vi "ConfigDialog-WithoutLoadingModules.vi"(8 "error in (no error)":errorcluster, 11 "INI File Path":path) -> (0 "error out":errorcluster)   [LabVIEW 2018]
uses:
  NistPluggableModules/Sensor/SensorPlugins/SensorBaseClass/SensorBase.lvclass
  C:/Program Files (x86)/National Instruments/LabVIEW 2018/user.lib/NIST/BaseClasses/BasePlugin_class/BasePlugin.lvclass
  <userlib>/NIST/BaseClasses/BasePlugin_class/BasePlugin.lvclass/BasePlugin.ctl
  <userlib>/NIST/ModuleAdminLib/CloneRegistration/CloneRegistration.lvclass
  <userlib>/NIST/ModuleAdminLib/ModuleAdmin/Accessors/Read CloneRegRef.vi
  <userlib>/NIST/BaseClasses/BasePlugin_class/Accessors/Write PluginIniFilePath.vi
  NistPluggableModules/Sync/SyncModule/Main.vi
  NistPluggableModules/FGen/FgenModule/Main.vi
  NistPluggableModules/Analysis/AnalysisModule/Main.vi
  <vilib>/Utility/error.llb/Error Cluster From Error Code.vi
  <vilib>/ErrorRing/Error Ring.xnode
  <userlib>/NIST/ModuleAdminLib/ModuleAdmin/ModuleAdmin.lvclass
  NistPluggableModules/Sync/SyncModule/SyncModule.lvlib
  <userlib>/NIST/NISTErrorLib/NISTErrorLib.lvlib
  NistPluggableModules/FGen/FgenModule/FgenModule.lvlib
  NistPluggableModules/Digitizer/DigitizerModule/DigitizerModule.lvlib
  NistPluggableModules/Scope/ScopeModule/ScopeModule.lvlib
  NistPluggableModules/Scope/ScopeShared/ScopeShared.lvlib
  NistPluggableModules/Analysis/AnalysisModule/AnalysisModule.lvlib
  NistPluggableModules/AcPwr/AcPwrModule/AcPwrModule.lvlib
  NistPluggableModules/AcPwr/AcPwrShared/AcPwrShared.lvlib
panel:
  out "Changed":bool
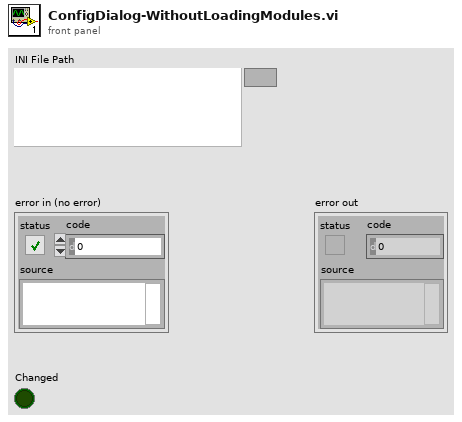
[diagram p1: front panel]
types:
  T1 = typedef "SyncModule.lvlib/clBroadcastEvents.ctl" = cluster{"DidInit":refnum<user-event>, "StatusUpdate":refnum<user-event>, "ErrorReport":refnum<user-event>, "DidStop":refnum<user-event>, "PathToINI":refnum<user-event>, "TriggerTime":refnum<user-event>, "LockStatus":refnum<user-event>, "Info":refnum<user-event>, "ClockProperties":refnum<user-event>}
  T2 = typedef "FgenModule.lvlib/clBroadcastEvents.ctl" = cluster{"DidInit":refnum<user-event>, "StatusUpdate":refnum<user-event>, "ErrorReport":refnum<user-event>, "DidStop":refnum<user-event>, "PathToINI":refnum<user-event>, "Channels":refnum<user-event>, "Function":refnum<user-event>, "Waveforms":refnum<user-event>, "Triggers":refnum<user-event>, "FunctionParams":refnum<user-event>, "FunctionArbs":refnum<user-event>, "FunctionSampleRate":refnum<user-event>}
  T3 = typedef "DigitizerShared.lvlib/clBroadcastEvents.ctl" = cluster{"DidInit":refnum<user-event>, "StatusUpdate":refnum<user-event>, "ErrorReport":refnum<user-event>, "DidStop":refnum<user-event>, "PathToINI":refnum<user-event>, "Channels":refnum<user-event>, "Acq":refnum<user-event>, "Trigger":refnum<user-event>, "Waveforms":refnum<user-event>}
  T4 = typedef "ScopeShared.lvlib/clBroadcastEvents.ctl" = cluster{"DidInit":refnum<user-event>, "StatusUpdate":refnum<user-event>, "ErrorReport":refnum<user-event>, "DidStop":refnum<user-event>, "PathToINI":refnum<user-event>, "Handle":refnum<user-event>, "Model":refnum<user-event>, "Channels":refnum<user-event>, "Acquisition":refnum<user-event>, "Trigger":refnum<user-event>, "ExtAcquisition":refnum<user-event>, "Waveform":refnum<user-event>}
  T5 = typedef "AnalysisModule.lvlib/clBroadcastEvents.ctl" = cluster{"DidInit":refnum<user-event>, "StatusUpdate":refnum<user-event>, "ErrorReport":refnum<user-event>, "DidStop":refnum<user-event>, "PathToINI":refnum<user-event>, "Config":refnum<user-event>, "ResultReport":refnum<user-event>, "FunctionClass":refnum<user-event>, "State":refnum<user-event>, "FunctionParams":refnum<user-event>, "Duration":refnum<user-event>}
  T6 = typedef "AcPwrShared.lvlib/AcPwrBroadcastEvents.ctl" = cluster{"DidInit":refnum<user-event>, "StatusUpdate":refnum<user-event>, "ErrorReport":refnum<user-event>, "DidStop":refnum<user-event>, "PathToINI":refnum<user-event>, "Measurements":refnum<user-event>, "LoadConfigFile":refnum<user-event>, "GetSettings":refnum<user-event>, "SetSettings":refnum<user-event>, "GetType&ID":refnum<user-event>, "GotSettings":refnum<user-event>}
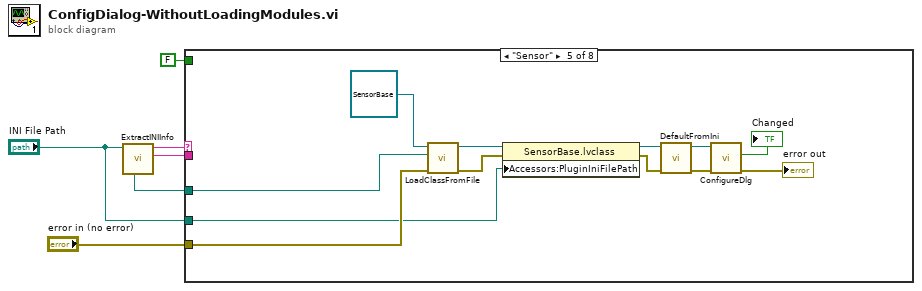
[diagram p0: block diagram]
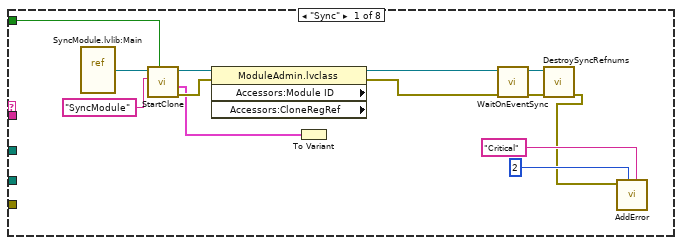
[diagram p2: hidden frame]
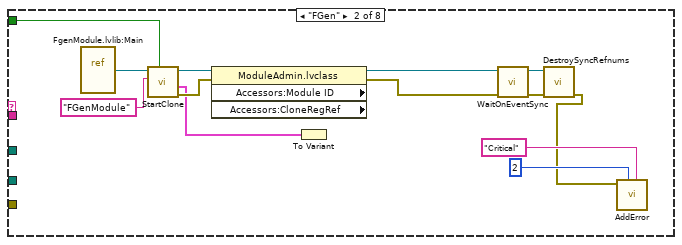
[diagram p3: hidden frame]
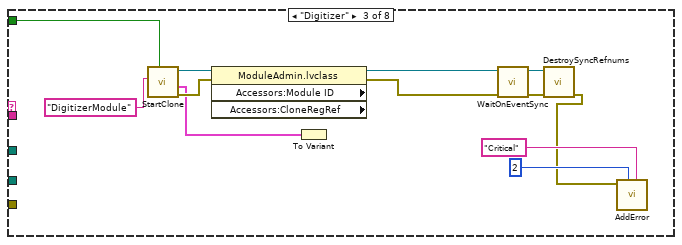
[diagram p4: hidden frame]
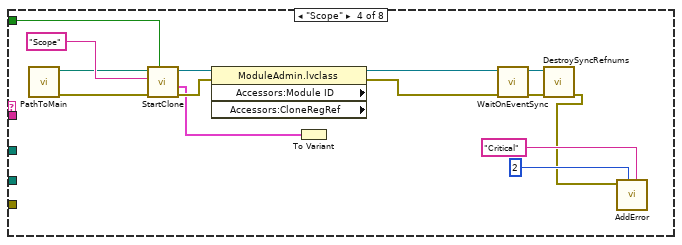
[diagram p5: hidden frame]
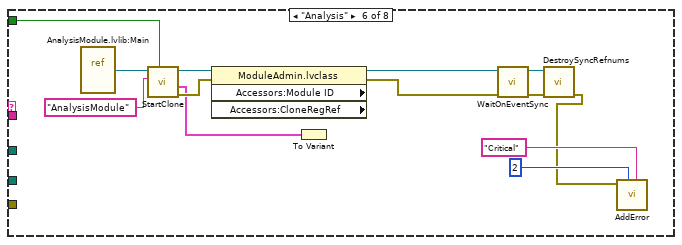
[diagram p6: hidden frame]
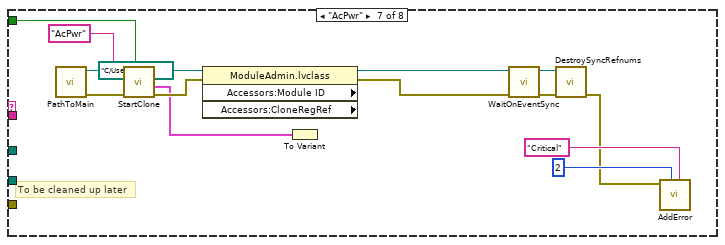
[diagram p7: hidden frame]
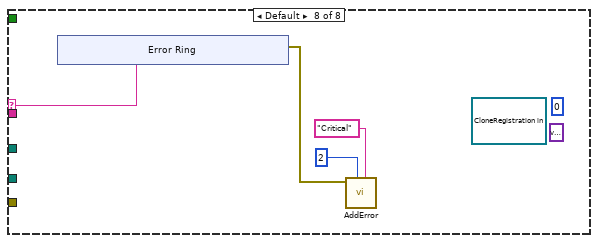
[diagram p8: hidden frame]
diagram:
  n1 = call "ExtractINIInfo.vi"("INI File Path"="INI File Path") -> ("Instrument name"=w4:string, "Module Name"=w6:string, "Instrument Class Path"=w1:path)  [unwired: 4 in, 4 out]
  n2 = case shown="\"Sensor\"" w6 {
    selector: w6 -> [_ _ _ _ _ _ _ w101]
    tunnel: FALSE ("ShowPanel? (f)") -> [w7 w20 w33 w47 _ w71 w86 _]
    tunnel: w4 -> [_ _ _ _ _ _ _ _]
    tunnel: "error in (no error)" -> [_ _ _ _ w68 _ _ _]
    tunnel: "INI File Path" -> [_ _ _ _ w65 _ _ _]
    tunnel: w1 -> [_ _ _ _ w59 _ _ _]
    frame "Sync" {
      n3 = vi-ref "SyncModule.lvlib:Main.vi"() -> (w19:refnum<vi>)
      n4 = call "StartClone.vi"("ShowPanel? (f)"=w7, "ModuleName"="SyncModule", "VI Refnum"=w19) -> ("error out"=w12:errorcluster, "SyncBroadcastEvents"=w11:T1, "ModuleAdmin"=w17:refnum<class "ModuleAdmin.lvclass">)  [unwired: 6 in]
      n5 = property class="ModuleAdmin.lvclass" props=["Accessors:Module ID", "Accessors:CloneRegRef"](reference=w17, error in=w12) -> (reference out=w15:refnum<class "ModuleAdmin.lvclass">, error out=w16:errorcluster)  [unwired: 2 out]
      n6 = To Variant(anything=w11) -> ()  [unwired: 1 out]
      n7 = call <userlib>:"WaitOnEventSync.vi"("error in (no error)"=w16, "ModuleAdmin"=w15) -> ("error out"=w14:errorcluster, "ModuleAdmin"=w13:refnum<class "ModuleAdmin.lvclass">)  [unwired: 8 in]
      n8 = call <userlib>:"DestroySyncRefnums.vi"("error in (no error)"=w14, "ModuleAdmin"=w13) -> ("error out"=w8:errorcluster)  [unwired: 9 in]
      n9 = call <userlib>:"AddError.vi"("Severity"="Critical", "Priority"=u8 2, "error in (no error)"=w8) -> ()  [unwired: 7 in, 2 out]
    }
    frame "FGen" {
      n10 = vi-ref "FgenModule.lvlib:Main.vi"() -> (w32:refnum<vi>)
      n11 = call "StartClone.vi"("ShowPanel? (f)"=w20, "ModuleName"="FGenModule", "VI Refnum"=w32) -> ("error out"=w25:errorcluster, "clBroadcastEvents"=w24:T2, "ModuleAdmin"=w30:refnum<class "ModuleAdmin.lvclass">)  [unwired: 6 in]
      n12 = property class="ModuleAdmin.lvclass" props=["Accessors:Module ID", "Accessors:CloneRegRef"](reference=w30, error in=w25) -> (reference out=w28:refnum<class "ModuleAdmin.lvclass">, error out=w29:errorcluster)  [unwired: 2 out]
      n13 = To Variant(anything=w24) -> ()  [unwired: 1 out]
      n14 = call <userlib>:"WaitOnEventSync.vi"("error in (no error)"=w29, "ModuleAdmin"=w28) -> ("error out"=w27:errorcluster, "ModuleAdmin"=w26:refnum<class "ModuleAdmin.lvclass">)  [unwired: 8 in]
      n15 = call <userlib>:"DestroySyncRefnums.vi"("error in (no error)"=w27, "ModuleAdmin"=w26) -> ("error out"=w21:errorcluster)  [unwired: 9 in]
      n16 = call <userlib>:"AddError.vi"("Severity"="Critical", "Priority"=u8 2, "error in (no error)"=w21) -> ()  [unwired: 7 in, 2 out]
    }
    frame "Digitizer" {
      n17 = call "StartClone.vi"("ShowPanel? (f)"=w33, "ModuleName"="DigitizerModule") -> ("error out"=w38:errorcluster, "clBroadcastEvents"=w37:T3, "ModuleAdmin"=w43:refnum<class "ModuleAdmin.lvclass">)  [unwired: 7 in]
      n18 = property class="ModuleAdmin.lvclass" props=["Accessors:Module ID", "Accessors:CloneRegRef"](reference=w43, error in=w38) -> (reference out=w41:refnum<class "ModuleAdmin.lvclass">, error out=w42:errorcluster)  [unwired: 2 out]
      n19 = To Variant(anything=w37) -> ()  [unwired: 1 out]
      n20 = call <userlib>:"WaitOnEventSync.vi"("error in (no error)"=w42, "ModuleAdmin"=w41) -> ("error out"=w40:errorcluster, "ModuleAdmin"=w39:refnum<class "ModuleAdmin.lvclass">)  [unwired: 8 in]
      n21 = call <userlib>:"DestroySyncRefnums.vi"("error in (no error)"=w40, "ModuleAdmin"=w39) -> ("error out"=w34:errorcluster)  [unwired: 9 in]
      n22 = call <userlib>:"AddError.vi"("Severity"="Critical", "Priority"=u8 2, "error in (no error)"=w34) -> ()  [unwired: 7 in, 2 out]
    }
    frame "Scope" {
      n23 = call "PathToMain.vi"() -> ("Error Out"=w46:errorcluster, "PathToMain"=w45:path)  [unwired: 10 in]
      n24 = call "StartClone.vi"("ShowPanel? (f)"=w47, "error in (no error)"=w46, "ModuleName"="Scope", "vi path"=w45) -> ("error out"=w52:errorcluster, "clBroadcastEvents"=w51:T4, "ModuleAdmin"=w57:refnum<class "ModuleAdmin.lvclass">)  [unwired: 5 in]
      n25 = property class="ModuleAdmin.lvclass" props=["Accessors:Module ID", "Accessors:CloneRegRef"](reference=w57, error in=w52) -> (reference out=w55:refnum<class "ModuleAdmin.lvclass">, error out=w56:errorcluster)  [unwired: 2 out]
      n26 = To Variant(anything=w51) -> ()  [unwired: 1 out]
      n27 = call <userlib>:"WaitOnEventSync.vi"("error in (no error)"=w56, "ModuleAdmin"=w55) -> ("error out"=w54:errorcluster, "ModuleAdmin"=w53:refnum<class "ModuleAdmin.lvclass">)  [unwired: 8 in]
      n28 = call <userlib>:"DestroySyncRefnums.vi"("error in (no error)"=w54, "ModuleAdmin"=w53) -> ("error out"=w48:errorcluster)  [unwired: 9 in]
      n29 = call <userlib>:"AddError.vi"("Severity"="Critical", "Priority"=u8 2, "error in (no error)"=w48) -> ()  [unwired: 7 in, 2 out]
    }
    frame "Sensor" {
      n30 = call-dynamic "LoadClassFromFile.vi"("error in (no error)"=w68, "class path"=w59, "reference in"=refnum<class "SensorBase.lvclass"> refnum ("SensorPlugins.lvlib:SensorBase.lvclass")) -> ("error out"=w69:errorcluster, "reference out"=w66:refnum<class "SensorBase.lvclass">)  [unwired: 7 in]
      n31 = property class="SensorBase.lvclass"(reference=w66, error in=w69, "Accessors:PluginIniFilePath"=w65) -> (reference out=w64:refnum<class "SensorBase.lvclass">, error out=w61:errorcluster)
      n32 = call-dynamic "DefaultFromIni.vi"("error in (no error)"=w61, "SensorBase in"=w64) -> ("error out"=w62:errorcluster, "SensorBase out"=w63:refnum<class "SensorBase.lvclass">)  [unwired: 8 in]
      n33 = call-dynamic "ConfigureDlg.vi"("error in (no error)"=w62, "PmuBase in"=w63) -> ("error out"=→"error out":errorcluster, "Changed"=→"Changed":bool)  [unwired: 7 in, 1 out]
    }
    frame "Analysis" {
      n34 = vi-ref "AnalysisModule.lvlib:Main.vi"() -> (w83:refnum<vi>)
      n35 = call "StartClone.vi"("ShowPanel? (f)"=w71, "ModuleName"="AnalysisModule", "VI Refnum"=w83) -> ("error out"=w76:errorcluster, "AnalysisBroadcastEvents"=w75:T5, "ModuleAdmin"=w81:refnum<class "ModuleAdmin.lvclass">)  [unwired: 6 in]
      n36 = property class="ModuleAdmin.lvclass" props=["Accessors:Module ID", "Accessors:CloneRegRef"](reference=w81, error in=w76) -> (reference out=w79:refnum<class "ModuleAdmin.lvclass">, error out=w80:errorcluster)  [unwired: 2 out]
      n37 = To Variant(anything=w75) -> ()  [unwired: 1 out]
      n38 = call <userlib>:"WaitOnEventSync.vi"("error in (no error)"=w80, "ModuleAdmin"=w79) -> ("error out"=w78:errorcluster, "ModuleAdmin"=w77:refnum<class "ModuleAdmin.lvclass">)  [unwired: 8 in]
      n39 = call <userlib>:"DestroySyncRefnums.vi"("error in (no error)"=w78, "ModuleAdmin"=w77) -> ("error out"=w72:errorcluster)  [unwired: 9 in]
      n40 = call <userlib>:"AddError.vi"("Severity"="Critical", "Priority"=u8 2, "error in (no error)"=w72) -> ()  [unwired: 7 in, 2 out]
    }
    frame "AcPwr" {
      (unwired) path "C:/Users/ico/Documents/Projects/NistPluggableModules/AcPwr/AcPwrPlugins/Common/Main.vi" ("vi path")
      # "To be cleaned up later"
      n41 = call "PathToMain.vi"() -> ("Error Out"=w85:errorcluster, "PathToMain"=w84:path)  [unwired: 10 in]
      n42 = call "StartClone.vi"("ShowPanel? (f)"=w86, "error in (no error)"=w85, "ModuleName"="AcPwr", "vi path"=w84) -> ("error out"=w91:errorcluster, "clAcPwrEvents"=w90:T6, "ModuleAdmin"=w96:refnum<class "ModuleAdmin.lvclass">)  [unwired: 5 in]
      n43 = property class="ModuleAdmin.lvclass" props=["Accessors:Module ID", "Accessors:CloneRegRef"](reference=w96, error in=w91) -> (reference out=w94:refnum<class "ModuleAdmin.lvclass">, error out=w95:errorcluster)  [unwired: 2 out]
      n44 = To Variant(anything=w90) -> ()  [unwired: 1 out]
      n45 = call <userlib>:"WaitOnEventSync.vi"("error in (no error)"=w95, "ModuleAdmin"=w94) -> ("error out"=w93:errorcluster, "ModuleAdmin"=w92:refnum<class "ModuleAdmin.lvclass">)  [unwired: 8 in]
      n46 = call <userlib>:"DestroySyncRefnums.vi"("error in (no error)"=w93, "ModuleAdmin"=w92) -> ("error out"=w87:errorcluster)  [unwired: 9 in]
      n47 = call <userlib>:"AddError.vi"("Severity"="Critical", "Priority"=u8 2, "error in (no error)"=w87) -> ()  [unwired: 7 in, 2 out]
    }
    frame Default {
      (unwired) variant ("Variant")
      (unwired) refnum<data-value> refnum ("Accessors:CloneRegRef")
      (unwired) 0 ("Accessors:Module ID")
      n48 = xnode "Error Ring"("parameter 0"=w101) -> ("error out"=w100:errorcluster)
      n49 = call <userlib>:"AddError.vi"("Severity"="Critical", "Priority"=u8 2, "error in (no error)"=w100) -> ()  [unwired: 7 in, 2 out]
    }
  }
